vi "Vision Processing.vi"(4 "error in (no error)":errorcluster, 7 "Image Size":T3=enum."320x240") -> ()   [LabVIEW 2015]
uses:
  Vision Support Code/Camera Types.ctl
  <vilib>/Rock Robotics/WPI/Camera/WPI_CameraImageSize.ctl
  <vilib>/Rock Robotics/WPI/Camera/WPI_CameraWhite Balance Values.ctl
  <vilib>/Rock Robotics/WPI/Camera/WPI_CameraExposure Values.ctl
  <vilib>/Rock Robotics/WPI/Camera/WPI_CameraFrameRate.ctl
  Robot Global Data.vi
  <vilib>/vision/NI_Vision_Development_Module.lvlib
panel:
  in  "Exposure (%)":dbl=0.3
  out "Highest Avg Score":dbl
  in  "Min Score Threshold":i32=75
  out "Detected Targets":T1(array[cluster]) {"Normalized Rect"."Numeric 5" format="%#_2g"; "Normalized Rect"."Numeric 3" format="%#_2g"; "Normalized Rect"."Numeric 2" format="%#_2g"; "Normalized Rect"."Numeric" format="%#_2g"}
  out "Sorted Particle Scores":T2(array[cluster]) {"Moment Factor" format="%#_3g"; "Aspect Ratio" format="%#_3g"; "Area to CH" format="%#_3g"; "X" format="%#_3g"; "Y" format="%#_3g"}
  in  "Display Original":bool=TRUE
  in  "Display Mask":bool=TRUE
  out "fps":dbl
  in  "Emphasize Limit Tests":bool=TRUE
  in  "Camera Type":T4=enum."MS HD3000 square"
  in  "Aspect Fudge Factor":dbl=1.0
  in  "Score Threshold":dbl=75.0
  out "ms to process":u32
  out "Qualified Particles":i32
  in  "LED Color":T5={"Hue"={180.0, 25.0}, "Sat"={66.78571428571429, 255.0}, "Val"={48.571428571428584, 255.0}} {"Hue" scale=0.0..255.0 scale format="%#_3g"}
  out "Masked":T6(plugin-control)
  out "Original Image":T6(plugin-control)
  # "This is only the initial camera size.\nOther camera setup is done\non the diagram. Notice it is set\nonce before the loop but can be\nupdated within the loop if needed."
  # "Instructions:\nUse LED Color to threshold and build particles. Adjust calibration if needed.\nDisplays are very useful for debugging, but will slow down execution, so you\nmay want to disable once working.\nAnnotations show the rectangle and the scores from top to bottom.\nChange camera setting on diagram."
  # "Density Profile"
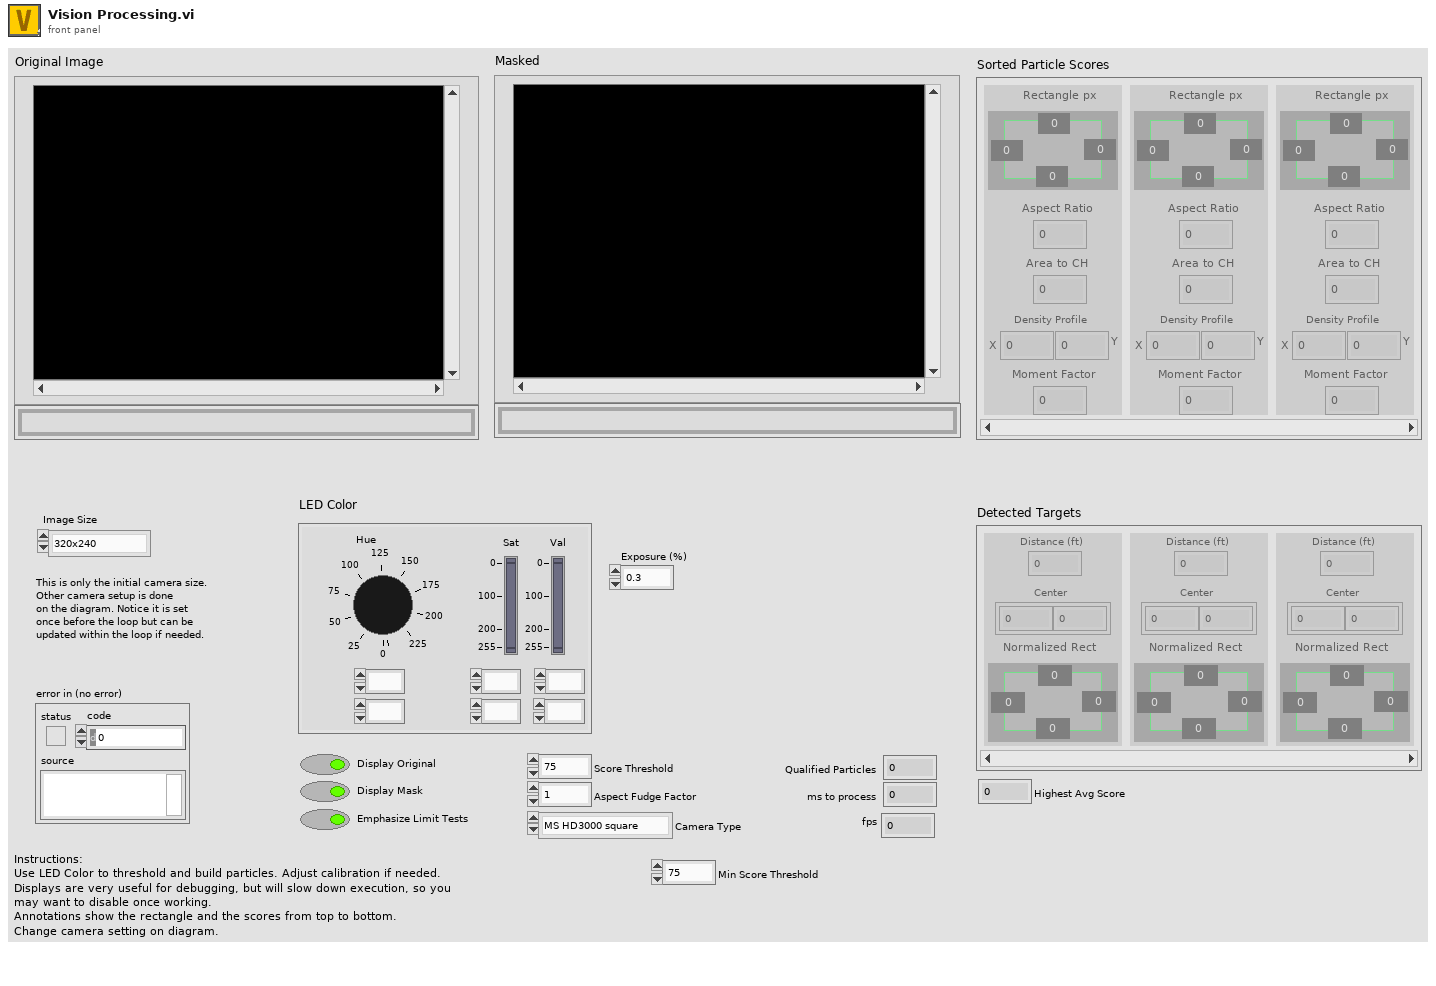
[diagram p1: front panel]
types:
  T1 = cluster{"Distance (ft)":dbl, "Center":cluster{dbl, dbl}, "Normalized Rect":cluster{"Numeric":dbl, "Numeric 2":dbl, "Numeric 3":dbl, "Numeric 5":dbl}}[]
  T2 = cluster{"Rectangle px":cluster{"Numeric":dbl, "Numeric 2":dbl, "Numeric 3":dbl, "Numeric 5":dbl}, "Aspect Ratio":dbl, "Area to CH":dbl, "X":dbl, "Y":dbl, "Moment Factor":dbl}[]
  T3 = typedef "WPI_CameraImageSize.ctl" = enum16{"640x480", "320x240", "160x120", "Custom"}
  T4 = typedef "Camera Types.ctl" = enum16{"206", "1011", "1013", "MS HD3000 square", "MS HD3000 640x480"}
  T5 = cluster{"Hue":cluster{dbl, dbl}, "Sat":cluster{dbl, dbl}, "Val":cluster{dbl, dbl}}
  T6 = typedef "IMAQ Image.ctl" = refnum<image>
  T7 = typedef "WPI_CameraFrameRate.ctl" = u32
  T8 = typedef "WPI_CameraExposure Values.ctl" = enum16{"Auto", "Flicker-free 50 Hz", "Flicker-free 60 Hz", "Hold current", "Custom"}
  T9 = typedef "WPI_CameraWhite Balance Values.ctl" = enum16{"Auto", "Fixed indoor", "Fixed outdoor 1", "Fixed outdoor 2", "Fixed fluorescent 1", "Fixed fluorescent 2", "Hold current", "Custom"}
  T10 = typedef "Particle Parameters" = i32
  T11 = typedef "Image Type" = u32
  T12 = typedef "WPI_CameraDevRef.ctl" = cluster{"Camera Address":string, "CameraStatus":errorcluster}
  T13 = cluster{"Bounding box":cluster{"left":dbl, "top":dbl, "right":dbl, "bottom":dbl}, "Aspect Ratio":dbl, "Area to CH":dbl, "X Mask":dbl, "Y Mask":dbl, "Moment":dbl}[]
  T14 = cluster{"Rectangle":cluster{"Numeric":dbl, "Numeric 2":dbl, "Numeric 3":dbl, "Numeric 5":dbl}, "L":dbl, "Area to CH":dbl, "X":dbl, "Y":dbl, "Moment Factor":dbl}[]
  T15 = cluster{"Rectangle":cluster{"Numeric":dbl, "Numeric 2":dbl, "Numeric 3":dbl, "Numeric 5":dbl}, "L":dbl, "Area to CH":dbl, "X":dbl, "Y":dbl, "Moment Factor":dbl}
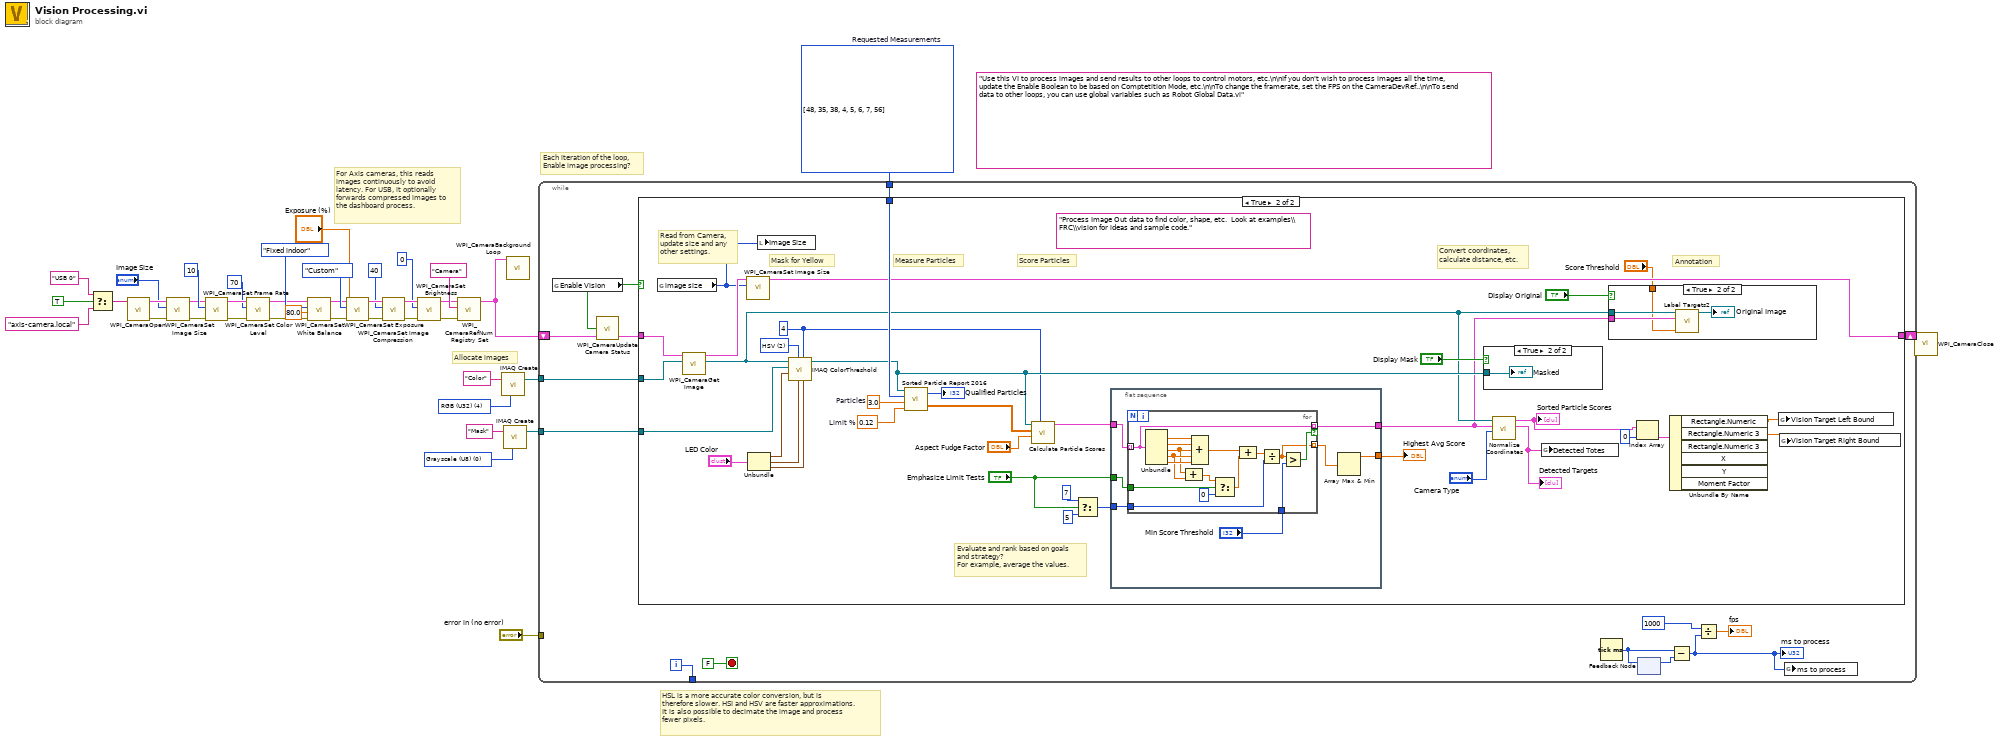
[diagram p0: block diagram]
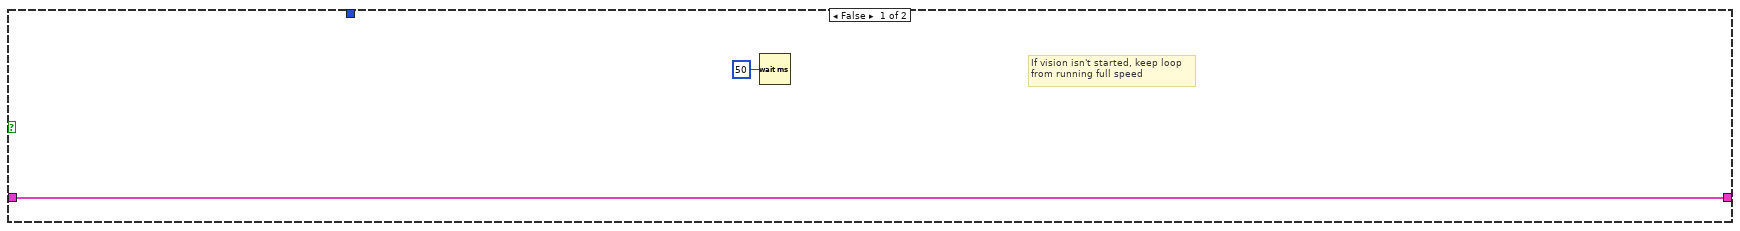
[diagram p2: hidden frame]
diagram:
  (unwired) "Use this VI to process images and send results to other loops to control motors, etc.\n\nIf you don't wish to process images all the time, update the Enable Boolean to be based on Comptetition Mode, etc.\n\nTo change the framerate, set the FPS on the CameraDevRef..\n\nTo send data to other loops, you can use global variables such as Robot Global Data.vi"
  w34 = T10[] [48, 35, 38, 4, 5, 6, 7, 56] items=["Center of Mass X", "Center of Mass Y", "First Pixel X", "First Pixel Y", "Bounding Rect Left", "Bounding Rect Top", "Bounding Rect Right", "Bounding Rect Bottom", "Max Feret Diameter Start X", "Max Feret Diameter Start Y", "Max Feret Diameter End X", "Max Feret Diameter End Y", "Max Horiz. Segment Length Left", "Max Horiz. Segment Length Right", "Max Horiz. Segment Length Row", "-", "Bounding Rect Width", "Bounding Rect Height", "Bounding Rect Diagonal", "Perimeter", "Convex Hull Perimeter", "Holes' Perimeter", "Max Feret Diameter", "Equivalent Ellipse Major Axis", "Equivalent Ellipse Minor Axis", "Equivalent Ellipse Minor Axis (Feret)", "Equivalent Rect Long Side", "Equivalent Rect Short Side", "Equivalent Rect Diagonal", "Equivalent Rect Short Side (Feret)", "Average Horiz. Segment Length", "Average Vert. Segment Length", "Hydraulic Radius", "Waddel Disk Diameter", "-", "Area", "Holes' Area", "Particle & Holes' Area", "Convex Hull Area", "Image Area", "-", "Number of Holes", "Number of Horiz. Segments", "Number of Vert. Segments", "-", "Orientation", "Max Feret Diameter Orientation", "-", "% Area/Image Area", "% Area/(Particle & Holes' Area)", "Ratio of Equivalent Ellipse Axes", "Ratio of Equivalent Rect Sides", "-", "Elongation Factor", "Compactness Factor", "Heywood Circularity Factor", "Type Factor", "-", "Sum X", "Sum Y", "Sum XX", "Sum XY", "Sum YY", "Sum XXX", "Sum XXY", "Sum XYY", "Sum YYY", "-", "Moment of Inertia XX", "Moment of Inertia XY", "Moment of Inertia YY", "Moment of Inertia XXX", "Moment of Inertia XXY", "Moment of Inertia XYY", "Moment of Inertia YYY", "Norm. Moment of Inertia XX", "Norm. Moment of Inertia XY", "Norm. Moment of Inertia YY", "Norm. Moment of Inertia XXX", "Norm. Moment of Inertia XXY", "Norm. Moment of Inertia XYY", "Norm. Moment of Inertia YYY", "Hu Moment 1", "Hu Moment 2", "Hu Moment 3", "Hu Moment 4", "Hu Moment 5", "Hu Moment 6", "Hu Moment 7"]  # Requested Measurements
  w37 = T11 0 items=["Grayscale (U8)", "Grayscale (I16)", "Grayscale (SGL)", "Complex (CSG)", "RGB (U32)", "HSL (U32)", "RGB (U64)", "Grayscale (U16)"] ("Image Type")
  w39 = T11 4 items=["Grayscale (U8)", "Grayscale (I16)", "Grayscale (SGL)", "Complex (CSG)", "RGB (U32)", "HSL (U32)", "RGB (U64)", "Grayscale (U16)"] ("Image Type")
  # "Each iteration of the loop,\nEnable image processing?"
  # "HSL is a more accurate color conversion, but is\ntherefore slower. HSI and HSV are faster approximations.\nIt is also possible to decimate the image and process\nfewer pixels."
  # "For Axis cameras, this reads\nimages continuously to avoid\nlatency. For USB, it optionally\nforwards compressed images to\nthe dashboard process."
  # "Allocate images"
  n1 = Select(t="USB 0" ("format string"), s=TRUE ("dot notation? (F)"), f="axis-camera.local" ("format string")) -> (s? t:f=w33:string)
  n2 = call <vilib>:"WPI_CameraOpen.vi"("Camera Address"=w33) -> ("error out"=w22:errorcluster, "CameraDevRef"=w21:T12)  [unwired: 1 in, 8 out]
  n3 = call <vilib>:"WPI_CameraSet Image Size.vi"("error in (no error)"=w22, "Image Size"="Image Size", "CameraDevRef"=w21) -> ("error out"=w23:errorcluster, "CameraDevRef Out"=w20:T12)  [unwired: 1 in, 6 out]
  n4 = call <vilib>:"WPI_CameraSet Frame Rate.vi"("error in (no error)"=w23, "Frame Rate (fps)"=T7 10, "CameraDevRef"=w20) -> ("error out"=w6:errorcluster, "CameraDevRef Out"=w7:T12)  [unwired: 7 out]
  n5 = call <vilib>:"WPI_CameraSet Color Level.vi"("error in (no error)"=w6, "Color Level"=70, "CameraDevRef"=w7) -> ("error out"=w4:errorcluster, "CameraDevRef Out"=w5:T12)  [unwired: 7 in]
  n6 = call <vilib>:"WPI_CameraSet White Balance.vi"("error in (no error)"=w4, "Color Temp (K)"=80.0, "White Balance"=WPI_CameraWhite_Balance_Values."Fixed indoor", "CameraDevRef"=w5) -> ("error out"=w24:errorcluster, "CameraDevRef Out"=w19:T12)  [unwired: 6 out]
  n7 = call <vilib>:"WPI_CameraSet Exposure.vi"("error in (no error)"=w24, "Exposure (%)"="Exposure (%)", "Exposure"=WPI_CameraExposure_Values."Custom", "CameraDevRef"=w19) -> ("error out"=w25:errorcluster, "CameraDevRef Out"=w17:T12)  [unwired: 6 out]
  n8 = call <vilib>:"WPI_CameraSet Image Compression.vi"("error in (no error)"=w25, "Compression"=40, "CameraDevRef"=w17) -> ("error out"=w26:errorcluster, "CameraDevRef Out"=w18:T12)  [unwired: 7 out]
  n9 = call <vilib>:"WPI_CameraSet Brightness.vi"("error in (no error)"=w26, "Brightness"=0, "CameraDevRef"=w18) -> ("error out"=w27:errorcluster, "CameraDevRef Out"=w9:T12)  [unwired: 7 out]
  n10 = call <vilib>:"WPI_CameraRefNum Registry Set.vi"("error in (no error)"=w27, "refnum name"="Camera", "CameraDevRef"=w9) -> ("CameraDevRef"=w14:T12)  [unwired: 1 in, 7 out]
  n11 = call "IMAQ Create"("Image Name"="Color", "Image Type"=w39) -> ("New Image"=w38:T6)  [unwired: 2 in, 2 out]
  n12 = call "IMAQ Create"("Image Name"="Mask", "Image Type"=w37) -> ("New Image"=w35:T6)  [unwired: 2 in, 2 out]
  n13 = call <vilib>:"WPI_CameraBackground Loop.vi"("CameraDevRef"=w14) -> ()  [unwired: 11 in]
  n14 = while {
    tunnel: w38 -> [w49]
    tunnel: w35 -> [w53]
    tunnel: w34 -> [w52]
    tunnel: "error in (no error)" -> [_]
    tunnel: [w48] -> _
    shift-right: [w44] -> w10
    shift-left: w14 -> [w46]
    i -> [w48]
    stop <- FALSE stop-if-true
    n15 = global read "Robot Global Data.vi" "Enable Vision"() -> (w47:bool)
    n16 = call <vilib>:"WPI_CameraUpdate Camera Status.vi"("CameraDevRef In"=w46, "Enable Vision"=w47) -> ("CameraDevRef Out"=w45:T12)  [unwired: 3 in]
    n17 = case shown="True" w47 {
      tunnel: w53 -> [_ w93]
      tunnel: w52 -> [_ w89]
      tunnel: w45 -> [w55 w85]
      tunnel: w49 -> [_ w84]
      tunnel: [w55 w82] -> w44
      frame False {
        # "If vision isn't started, keep loop\nfrom running full speed"
        n18 = Wait (ms)(milliseconds to wait=u32 50) -> ()  [unwired: 1 out]
      }
      frame True {
        w66 = 4 ("Replace Value")
        w79 = u16 2 items=["RGB", "HSL", "HSV", "HSI"] ("Color Mode")
        (unwired) "Process Image Out data to find color, shape, etc.  Look at examples\\FRC\\vision for ideas and sample code."
        w86 = 0.12  # Limit %
        w88 = 3.0  # Particles
        # "Evaluate and rank based on goals\nand strategy?\nFor example, average the values."
        # "Read from Camera,\nupdate size and any\nother settings."
        # "Measure Particles"
        # "Convert coordinates,\ncalculate distance, etc."
        # "Annotation"
        # "Score Particles"
        # "Mask for Yellow"
        n19 = global read "Robot Global Data.vi" "image size"() -> (w64:T3)
        n20 = call <vilib>:"WPI_CameraGet Image.vi"("Image"=w84, "CameraDevRef"=w85) -> ("Image Out"=w69:T6, "CameraDevRef Out"=w83:T12)  [unwired: 7 in, 1 out]
        n21 = call <vilib>:"WPI_CameraSet Image Size.vi"("Image Size"=w64, "CameraDevRef"=w83) -> ("CameraDevRef Out"=w82:T12)  [unwired: 2 in, 7 out]
        n22 = Unbundle("LED Color") -> ("Hue"=w92:cluster{dbl, dbl}, "Sat"=w91:cluster{dbl, dbl}, "Val"=w90:cluster{dbl, dbl})
        n23 = local write "Image Size"(w64) -> ()
        n24 = call "IMAQ ColorThreshold"("Blue or Luma or Val or Inten Range"=w90, "Replace Value"=w66, "Green or Sat Range"=w91, "Color Mode"=w79, "Red or Hue Range"=w92, "Image Dst"=w93, "Image Src"=w69) -> ("Image Dst Out"=w78:T6)  [unwired: 3 in, 1 out]
        n25 = call "Sorted Particle Report 2016.vi"("Min Area Size %"=w86, "Particle Count Limit"=w88, "Pixel Measurements"=w89, "Image in"=w78) -> ("Sorted Data"=w77:dbl[][], "Particles"=→"Qualified Particles":i32)
        n26 = call "Calculate Particle Scores.vi"("Pixel Value"=w66, "Aspect Fudge Factor"="Aspect Fudge Factor", "Sorted Data"=w77, "Image in"=w78) -> ("Scores"=w75:T13)  [unwired: 7 in]
        n27 = Select(t=7, s="Emphasize Limit Tests", f=5) -> (s? t:f=w72:i32)
        n28 = flat-sequence {
          tunnel: w75 -> [w104]
          tunnel: w72 -> [w102]
          tunnel: [w105] -> w71
          tunnel: [w99] -> w68
          tunnel: "Emphasize Limit Tests" -> [w103]
          frame #0 {
            n29 = for {
              tunnel: w104 -> [w119] mode=indexing
              tunnel: [w119] -> w99 mode=indexing if=w118
              tunnel: [w117] -> w100 mode=indexing
              tunnel: w102 -> [w116]
              tunnel: "Min Score Threshold" -> [w115]
              tunnel: w103 -> [w108]
              n30 = Unbundle(w119) -> ("Aspect Ratio"=w121:dbl, "Area to CH"=w120:dbl, "X Mask"=w110:dbl, "Y Mask"=w111:dbl, "Moment"=w112:dbl)  [unwired: 1 out]
              n31 = Compound Arithmetic op=ADD(w110, w111) -> (w109:dbl)
              n32 = Compound Arithmetic op=ADD(w121, w120, w110, w111, w112) -> (w114:dbl)
              n33 = Select(t=w109, s=w108, f=0) -> (s? t:f=w107:dbl)
              n34 = Compound Arithmetic op=ADD(w114, w107) -> (w113:dbl)
              n35 = Divide(x=w113, y=w116) -> (x/y=w117:dbl)
              n36 = Greater?(x=w117, y=w115) -> (0:w118:bool)
            }
            n37 = Array Max & Min(array=w100) -> (max value=w105:dbl)  [unwired: 3 out]
          }
        }
        n38 = case shown="True" "Display Mask" {
          tunnel: w78 -> [_ w98]
          frame False {
          }
          frame True {
            "Masked" <- w98
          }
        }
        n39 = call "Normalize Coordinates.vi"("Camera Type"="Camera Type", "Targets"=w68, "Image in"=w69) -> ("Found Targets"=w65:T1, "Sorted Scores"=w61:T14)  [unwired: 7 in]
        "Sorted Particle Scores" <- w61
        "Detected Targets" <- w65
        n40 = global write "Robot Global Data.vi" "Detected Totes"(w65) -> ()
        n41 = case shown="True" "Display Original" {
          tunnel: w69 -> [_ w97]
          tunnel: w68 -> [_ w95]
          tunnel: "Score Threshold" -> [_ w94]
          frame False {
          }
          frame True {
            n42 = call "Label Targets2.vi"("Score Threshold"=w94, "Targets"=w95, "Image in"=w97) -> ("Image out"=→"Original Image":T6)  [unwired: 8 in]
          }
        }
        n43 = Index Array(array=w61, index=0) -> (element=w59:T15)
        n44 = Unbundle By Name(w59) -> ("Rectangle.Numeric"=w58:dbl, "Rectangle.Numeric 3"=w57:dbl)  [unwired: 4 out]
        n45 = global write "Robot Global Data.vi" "Vision Target Left Bound"(w58) -> ()
        n46 = global write "Robot Global Data.vi" "Vision Target Right Bound"(w57) -> ()
        "Highest Avg Score" <- w71
      }
    }
    n47 = Tick Count (ms)() -> (millisecond timer value=w50:u32)
    n48 = feedback-in #1(w50) -> ()
    n49 = feedback #1() -> (w51:u32)  [unwired: 1 in]
    n50 = Subtract(x=w50, y=w51) -> (x-y=w43:u32)
    "ms to process" <- w43
    n51 = Divide(x=1000 ("Brightness"), y=w43) -> (x/y=→"fps":dbl)
    n52 = global write "Robot Global Data.vi" "ms to process"(w43) -> ()
  }
  n53 = call <vilib>:"WPI_CameraClose.vi"("CameraDevRef"=w10) -> ()  [unwired: 1 in, 10 out]
